vi "Reset Device Core.vi"(8 "error in (no error)":errorcluster, 11 "KIT-QVA in":refnum<class "KIT-QVA.lvclass">) -> (0 "error out":errorcluster, 3 "KIT-QVA out":refnum<class "KIT-QVA.lvclass">)   [LabVIEW 2014, in "KIT-QVA.lvlib" / "KIT-QVA.lvclass"]
doc: "Perform reset of device."
uses:
  KIT-QVA.lvclass
  KIT-QVA.lvclass/KIT-QVA.ctl
  CSPP_Core/Actors/CS++DeviceActor/CS++DeviceActor.lvclass
  instr.lib/KIT-QV/KIT QV.lvlib
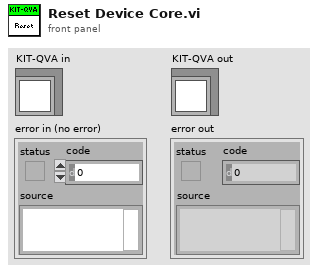
[diagram p1: front panel]
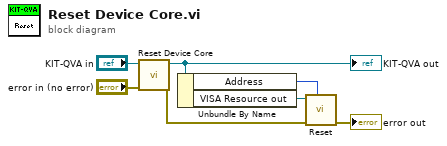
[diagram p0: block diagram]
diagram:
  n1 = call-parent "Reset Device Core.vi"("error in (no error)"="error in (no error)", "CS++DeviceActor in"="KIT-QVA in") -> ("error out"=w5:errorcluster, "CS++DeviceActor out"=w2:refnum<class "KIT-QVA.lvclass">)  [unwired: 8 in]
  "KIT-QVA out" <- w2
  n2 = Unbundle By Name(w2) -> ("Address"=w1:u16, "VISA Resource out"=w3:refnum<visa-resource-name>)
  n3 = call "Reset.vi"("Address"=w1, "Error In"=w5, "VISA Resource in"=w3) -> ("Error Out"=→"error out":errorcluster)  [unwired: 7 in, 1 out]
